vi "1.2.vi"() -> ()   [LabVIEW 2016]
panel:
  out "X/Y":dbl
  out "X+Y":dbl
  out "布尔":bool
  in  "Y":dbl
  in  "X":dbl
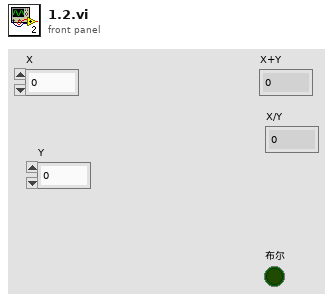
[diagram p1: front panel]
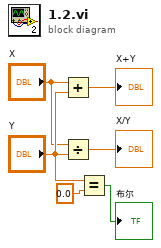
[diagram p0: block diagram]
diagram:
  n1 = Add(x="X", y="Y") -> (x+y=→"X+Y":dbl)
  n2 = Divide(x="X", y="Y") -> (x/y=→"X/Y":dbl)
  n3 = Equal?(x="Y", y=0.0) -> (x = y?=→"布尔":bool)
